vi "Initialize 8 NEO Swerve Drive.vi"() -> (0 "error out":errorcluster, 3 "Motors":T1={"Drive Motors (NEO)"={"Left Front"={"DeviceStatus"={"status"=FALSE, "code"=0, "source"=""}, "Type"=enum."PWM", "PWM"={"PWM Channel"=enum."Invalid", "DeadBand"={"Name"="", "maxPositivePwm"=0, "minPositivePwm"=0, "centerPwm"=0, "maxNegativePwm"=0, "minNegativePwm"=0, "angularRange"=0}}, "CAN"={"Device Number"=0, "SetOutput VI Ref"=variant, "GetOutput VI Ref"=variant, "Enable VI Ref"=variant, "Disable VI Ref"=variant, "Data"=variant}, "Invert"=FALSE, "DIO PWM"={"PWM \"Enable\" Channel"=enum."Invalid", "DIOChannel"=enum."Invalid", "PWM Rate"=0.0}}, "Left Back"={"DeviceStatus"={"status"=FALSE, "code"=0, "source"=""}, "Type"=enum."PWM", "PWM"={"PWM Channel"=enum."Invalid", "DeadBand"={"Name"="", "maxPositivePwm"=0, "minPositivePwm"=0, "centerPwm"=0, "maxNegativePwm"=0, "minNegativePwm"=0, "angularRange"=0}}, "CAN"={"Device Number"=0, "SetOutput VI Ref"=variant, "GetOutput VI Ref"=variant, "Enable VI Ref"=variant, "Disable VI Ref"=variant, "Data"=variant}, "Invert"=FALSE, "DIO PWM"={"PWM \"Enable\" Channel"=enum."Invalid", "DIOChannel"=enum."Invalid", "PWM Rate"=0.0}}, "Right Front"={"DeviceStatus"={"status"=FALSE, "code"=0, "source"=""}, "Type"=enum."PWM", "PWM"={"PWM Channel"=enum."Invalid", "DeadBand"={"Name"="", "maxPositivePwm"=0, "minPositivePwm"=0, "centerPwm"=0, "maxNegativePwm"=0, "minNegativePwm"=0, "angularRange"=0}}, "CAN"={"Device Number"=0, "SetOutput VI Ref"=variant, "GetOutput VI Ref"=variant, "Enable VI Ref"=variant, "Disable VI Ref"=variant, "Data"=variant}, "Invert"=FALSE, "DIO PWM"={"PWM \"Enable\" Channel"=enum."Invalid", "DIOChannel"=enum."Invalid", "PWM Rate"=0.0}}, "Right Back"={"DeviceStatus"={"status"=FALSE, "code"=0, "source"=""}, "Type"=enum."PWM", "PWM"={"PWM Channel"=enum."Invalid", "DeadBand"={"Name"="", "maxPositivePwm"=0, "minPositivePwm"=0, "centerPwm"=0, "maxNegativePwm"=0, "minNegativePwm"=0, "angularRange"=0}}, "CAN"={"Device Number"=0, "SetOutput VI Ref"=variant, "GetOutput VI Ref"=variant, "Enable VI Ref"=variant, "Disable VI Ref"=variant, "Data"=variant}, "Invert"=FALSE, "DIO PWM"={"PWM \"Enable\" Channel"=enum."Invalid", "DIOChannel"=enum."Invalid", "PWM Rate"=0.0}}}, "Steer Motors (NEO)"={"Left Front"={"DeviceStatus"={"status"=FALSE, "code"=0, "source"=""}, "Type"=enum."PWM", "PWM"={"PWM Channel"=enum."Invalid", "DeadBand"={"Name"="", "maxPositivePwm"=0, "minPositivePwm"=0, "centerPwm"=0, "maxNegativePwm"=0, "minNegativePwm"=0, "angularRange"=0}}, "CAN"={"Device Number"=0, "SetOutput VI Ref"=variant, "GetOutput VI Ref"=variant, "Enable VI Ref"=variant, "Disable VI Ref"=variant, "Data"=variant}, "Invert"=FALSE, "DIO PWM"={"PWM \"Enable\" Channel"=enum."Invalid", "DIOChannel"=enum."Invalid", "PWM Rate"=0.0}}, "Left Back"={"DeviceStatus"={"status"=FALSE, "code"=0, "source"=""}, "Type"=enum."PWM", "PWM"={"PWM Channel"=enum."Invalid", "DeadBand"={"Name"="", "maxPositivePwm"=0, "minPositivePwm"=0, "centerPwm"=0, "maxNegativePwm"=0, "minNegativePwm"=0, "angularRange"=0}}, "CAN"={"Device Number"=0, "SetOutput VI Ref"=variant, "GetOutput VI Ref"=variant, "Enable VI Ref"=variant, "Disable VI Ref"=variant, "Data"=variant}, "Invert"=FALSE, "DIO PWM"={"PWM \"Enable\" Channel"=enum."Invalid", "DIOChannel"=enum."Invalid", "PWM Rate"=0.0}}, "Right Front"={"DeviceStatus"={"status"=FALSE, "code"=0, "source"=""}, "Type"=enum."PWM", "PWM"={"PWM Channel"=enum."Invalid", "DeadBand"={"Name"="", "maxPositivePwm"=0, "minPositivePwm"=0, "centerPwm"=0, "maxNegativePwm"=0, "minNegativePwm"=0, "angularRange"=0}}, "CAN"={"Device Number"=0, "SetOutput VI Ref"=variant, "GetOutput VI Ref"=variant, "Enable VI Ref"=variant, "Disable VI Ref"=variant, "Data"=variant}, "Invert"=FALSE, "DIO PWM"={"PWM \"Enable\" Channel"=enum."Invalid", "DIOChannel"=enum."Invalid", "PWM Rate"=0.0}}, "Right Back"={"DeviceStatus"={"status"=FALSE, "code"=0, "source"=""}, "Type"=enum."PWM", "PWM"={"PWM Channel"=enum."Invalid", "DeadBand"={"Name"="", "maxPositivePwm"=0, "minPositivePwm"=0, "centerPwm"=0, "maxNegativePwm"=0, "minNegativePwm"=0, "angularRange"=0}}, "CAN"={"Device Number"=0, "SetOutput VI Ref"=variant, "GetOutput VI Ref"=variant, "Enable VI Ref"=variant, "Disable VI Ref"=variant, "Data"=variant}, "Invert"=FALSE, "DIO PWM"={"PWM \"Enable\" Channel"=enum."Invalid", "DIOChannel"=enum."Invalid", "PWM Rate"=0.0}}}, "Pigeon2"={"DeviceStatus"={"status"=FALSE, "code"=0, "source"=""}, "Device Number"=0, "Type"=352321536, "Device ID"=0, "Handle"=0, "UsageFrame"=0, "Library Path"=path ""}, "Radii (ft)"={"Left Front Position"=[], "Left Back Position"=[], "Right Front Position"=[], "Right Back Position"=[]}} {"Radii (ft)"."Right Back Position" format="%.2f"; "Radii (ft)"."Right Front Position" format="%.2f"; "Radii (ft)"."Left Back Position" format="%.2f"; "Radii (ft)"."Left Front Position" format="%.2f"; "Pigeon2"."Type" items=["CAN"=352321536, "TalonSRX"=33554432]})   [LabVIEW 2025]
doc: "Creates a cluster of 4 motors (order is left-front, left-back, right-front, right-back) initialized with PID coefficients and status frame reduction"
uses:
  <vilib>/Rock Robotics/WPI/ThirdParty/REV Robotics/REVLib/Typedef/Spark MAX Idle Mode.ctl
  <vilib>/Rock Robotics/WPI/MotorControl/WPI_MotorControlType.ctl
  <vilib>/Rock Robotics/SystemInterfaces/DIO/FPGA_DIOPWMChannel.ctl
  <vilib>/Rock Robotics/WPI/PWM/WPI_PWMDeadband.ctl
  <vilib>/Rock Robotics/SystemInterfaces/DIO/FPGA_DIOChannel.ctl
  <vilib>/Rock Robotics/WPI/MotorControl/WPI_MotorControlDeviceRef.ctl
  Type Definitions/Hardware/4 Motor Sets/(NEO & NEO 550) 4 Motor Set.ctl
  Type Definitions/Hardware/Swerve Drives/(NEO-NEO-ThroughBore-Pigeon2) Swerve.ctl
  Type Definitions/Data/Pod Positions.ctl
  <vilib>/Rock Robotics/WPI/ThirdParty/Phoenix-LabVIEW/Pigeon IMU/CTRE_PigeonIMU_ConnectionType.ctl
  <vilib>/Rock Robotics/WPI/ThirdParty/Phoenix-LabVIEW/Pigeon IMU/CTRE_PigeonIMU_DeviceRef.ctl
  Type Definitions/Hardware/Swerve Configs/NEO-NEO-ThroughBore-Pigeon2 Swerve Config.ctl
  <vilib>/Rock Robotics/WPI/ThirdParty/REV Robotics/REVLib/SubVI/Public/SPARK Open Brushless.vi
  <vilib>/Rock Robotics/WPI/ThirdParty/REV Robotics/REVLib/Typedef/Spark MAX Status Frames.ctl
  <vilib>/Rock Robotics/WPI/ThirdParty/REV Robotics/REVLib/Typedef/Closed Loop Voltage Mode.ctl
  <vilib>/Rock Robotics/WPI/ThirdParty/REV Robotics/REVLib/Typedef/SPARK Feedback Sensor.ctl
  <vilib>/Rock Robotics/WPI/ThirdParty/REV Robotics/REVLib/SubVI/Public/SPARK Configure Encoder Conversion Factors.vi
  <vilib>/Rock Robotics/WPI/ThirdParty/REV Robotics/REVLib/SubVI/Public/SPARK Configure Power Smart Current Limit.vi
  <vilib>/Rock Robotics/WPI/ThirdParty/REV Robotics/REVLib/SubVI/Public/SPARK Configure Basic Idle Mode.vi
  <vilib>/Rock Robotics/WPI/ThirdParty/REV Robotics/REVLib/SubVI/Public/SPARK Configure Closed Loop Voltage Mode.vi
  <vilib>/Rock Robotics/WPI/ThirdParty/REV Robotics/REVLib/SubVI/Public/SPARK Configure Closed Loop Basic.vi
  <vilib>/Rock Robotics/WPI/ThirdParty/REV Robotics/REVLib/SubVI/Public/SPARK Configure Closed Loop Position Wrapping.vi
  <vilib>/Rock Robotics/WPI/ThirdParty/REV Robotics/REVLib/SubVI/Public/SPARK Configure Encoder Velocity Filtering UVW.vi
  <vilib>/Rock Robotics/WPI/ThirdParty/REV Robotics/REVLib/Typedef/Spark MAX Hall Sensor Average Depth Size.ctl
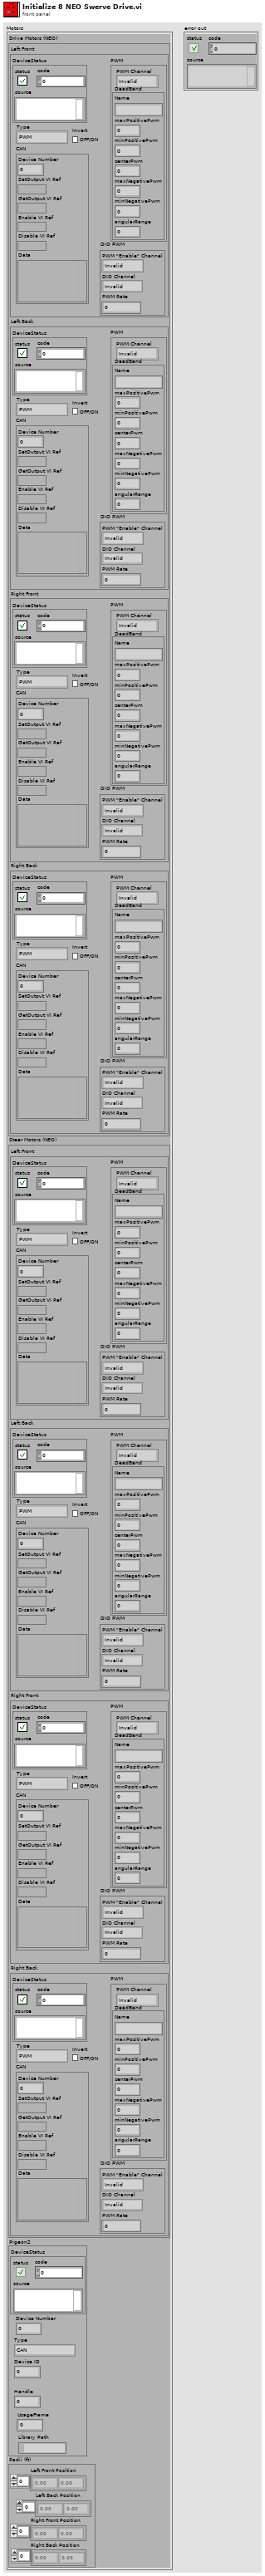
[diagram p1: front panel]
types:
  T1 = typedef "(NEO-NEO-ThroughBore-Pigeon2) Swerve.ctl" = cluster{"Drive Motors (NEO)":T2, "Steer Motors (NEO)":T2, "Pigeon2":T8, "Radii (ft)":T10}
  T2 = typedef "(NEO & NEO 550) 4 Motor Set.ctl" = cluster{"Left Front":T3, "Left Back":T3, "Right Front":T3, "Right Back":T3}
  T3 = typedef "WPI_MotorControlDeviceRef.ctl" = cluster{"DeviceStatus":errorcluster, "Type":T4, "PWM":cluster{"PWM Channel":T5, "DeadBand":T6}, "CAN":cluster{"Device Number":u8, "SetOutput VI Ref":variant, "GetOutput VI Ref":variant, "Enable VI Ref":variant, "Disable VI Ref":variant, "Data":variant}, "Invert":bool, "DIO PWM":cluster{"PWM \"Enable\" Channel":T5, "DIOChannel":T7, "PWM Rate":dbl}}
  T4 = typedef "WPI_MotorControlType.ctl" = enum16{"PWM", "CAN", "DIO PWM"}
  T5 = typedef "FPGA_DIOPWMChannel.ctl" = enum8{"PWM 0", "PWM 1", "PWM 2", "PWM 3", "PWM 4", "PWM 5", "PWM 6", "PWM 7", "PWM 8", "PWM 9", "PWM MXP 0", "PWM MXP 1", "PWM MXP 2", "PWM MXP 3", "PWM MXP 4", "PWM MXP 5", "PWM MXP 6", "PWM MXP 7", "PWM MXP 8", "PWM MXP 9", "Invalid"}
  T6 = typedef "WPI_PWMDeadband.ctl" = cluster{"Name":string, "maxPositivePwm":i32, "minPositivePwm":i32, "centerPwm":i32, "maxNegativePwm":i32, "minNegativePwm":i32, "angularRange":u16}
  T7 = typedef "FPGA_DIOChannel.ctl" = enum8{"DIO 0", "DIO 1", "DIO 2", "DIO 3", "DIO 4", "DIO 5", "DIO 6", "DIO 7", "DIO 8", "DIO 9", "DIO MXP 0", "DIO MXP 1", "DIO MXP 2", "DIO MXP 3", "DIO MXP 4", "DIO MXP 5", "DIO MXP 6", "DIO MXP 7", "DIO MXP 8", "DIO MXP 9", "DIO MXP 10", "DIO MXP 11", "DIO MXP 12", "DIO MXP 13", "DIO MXP 14", "DIO MXP 15", "SPI Port CS1", "SPI Port CS2", "SPI Port CS3", "SPI Port MISO", "SPI Port MOSI", "Invalid"}
  T8 = typedef "CTRE_PigeonIMU_DeviceRef.ctl" = cluster{"DeviceStatus":errorcluster, "Device Number":u8, "Type":T9, "Device ID":u32, "Handle":u64, "UsageFrame":u32, "Library Path":path}
  T9 = typedef "CTRE_PigeonIMU_ConnectionType.ctl" = u32
  T10 = typedef "Pod Positions.ctl" = cluster{"Left Front Position":dbl[], "Left Back Position":dbl[], "Right Front Position":dbl[], "Right Back Position":dbl[]}
  T11 = typedef "NEO-NEO-ThroughBore-Pigeon2 Swerve Config.ctl" = cluster{"Drive Motor CAN IDs":cluster{"LF CAN ID":dbl, "LB CAN ID":dbl, "RF CAN ID":dbl, "RB CAN ID":dbl}, "Steer Motor CAN IDs":cluster{"LF CAN ID":dbl, "LB CAN ID":dbl, "RF CAN ID":dbl, "RB CAN ID":dbl}, "Drive PID Constants":cluster{"P Gain":dbl, "I Gain":dbl, "D Gain":dbl, "F Gain":dbl, "I Zone":dbl, "Min Output":dbl, "Max Output":dbl}, "Steer PID Constants":cluster{"P Gain":dbl, "I Gain":dbl, "D Gain":dbl, "F Gain":dbl, "I Zone":dbl, "Min Output":dbl, "Max Output":dbl}, "Pigeon 2 Refnum":string, "Pod Locations (ft)":T10}
  T12 = cluster{"LF CAN ID":dbl, "LB CAN ID":dbl, "RF CAN ID":dbl, "RB CAN ID":dbl}
  T13 = cluster{"P Gain":dbl, "I Gain":dbl, "D Gain":dbl, "F Gain":dbl, "I Zone":dbl, "Min Output":dbl, "Max Output":dbl}
  T14 = typedef "Spark MAX Hall Sensor Average Depth Size.ctl" = enum16{"1", "2", "4", "8"}
  T15 = typedef "SPARK Feedback Sensor.ctl" = enum16{"No Sensor", "Primary Encoder", "Analog Sensor", "Alternate or External Encoder", "Duty Cycle Sensor"}
  T16 = typedef "Closed Loop Voltage Mode.ctl" = enum16{"Disabled", "Voltage Output", "Voltage Compensation"}
  T17 = typedef "Spark MAX Status Frames.ctl" = enum16{"Status 0", "Status 1", "Status 2", "Status 3", "Status 4", "Status 5", "Status 6", "Status 7"}
  T18 = typedef "Spark MAX Idle Mode.ctl" = enum16{"Coast", "Brake"}
  T19 = typedef "DeviceReference.ctl" = cluster{"CANbus Name":string, "Device Encoding":u32, "Device Name":string}
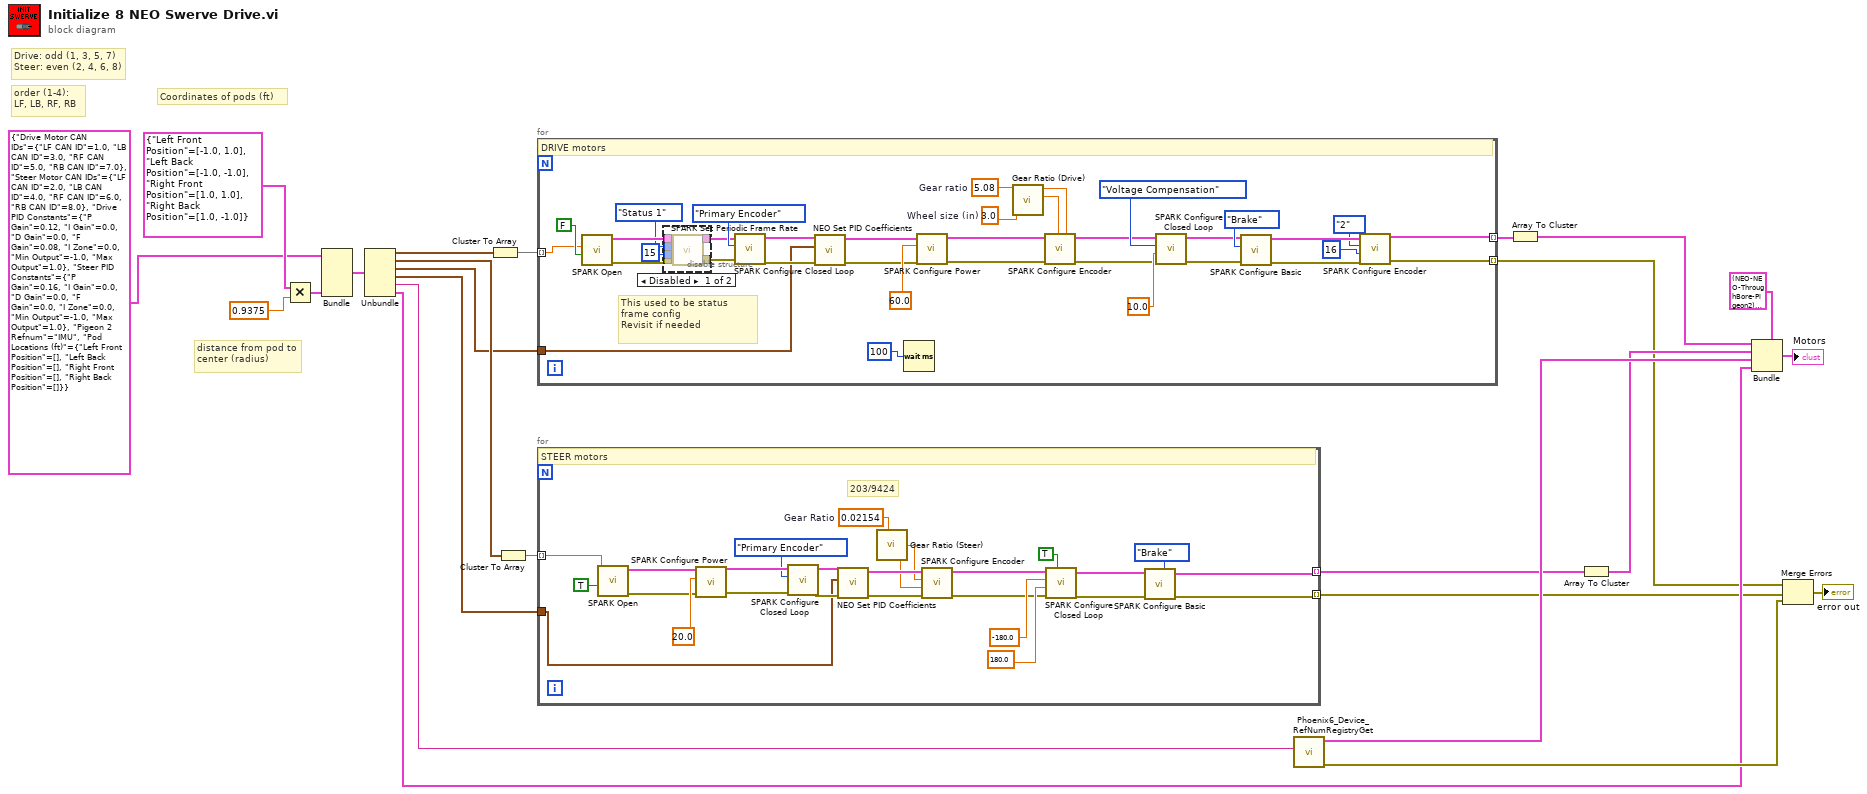
[diagram p0: block diagram]
diagram:
  # "Drive: odd (1, 3, 5, 7)\nSteer: even (2, 4, 6, 8)"
  # "Coordinates of pods (ft)"
  # "distance from pod to center (radius)"
  # "order (1-4):\nLF, LB, RF, RB"
  n1 = Multiply(x=T10 {"Left Front Position"=[-1.0, 1.0], "Left Back Position"=[-1.0, -1.0], "Right Front Position"=[1.0, 1.0], "Right Back Position"=[1.0, -1.0]} ("Radii (ft)"), y=0.9375 ("Pod Radius")) -> (x*y=w11:T10)
  n2 = Bundle(cluster=T11 {"Drive Motor CAN IDs"={"LF CAN ID"=1.0, "LB CAN ID"=3.0, "RF CAN ID"=5.0, "RB CAN ID"=7.0}, "Steer Motor CAN IDs"={"LF CAN ID"=2.0, "LB CAN ID"=4.0, "RF CAN ID"=6.0, "RB CAN ID"=8.0}, "Drive PID Constants"={"P Gain"=0.12, "I Gain"=0.0, "D Gain"=0.0, "F Gain"=0.08, "I Zone"=0.0, "Min Output"=-1.0, "Max Output"=1.0}, "Steer PID Constants"={"P Gain"=0.16, "I Gain"=0.0, "D Gain"=0.0, "F Gain"=0.0, "I Zone"=0.0, "Min Output"=-1.0, "Max Output"=1.0}, "Pigeon 2 Refnum"="IMU", "Pod Locations (ft)"={"Left Front Position"=[], "Left Back Position"=[], "Right Front Position"=[], "Right Back Position"=[]}} ("Swerve Config"), "Pod Locations (ft)"=w11) -> (w20:T11)  [unwired: 5 in]
  n3 = Unbundle(w20) -> ("Drive Motor CAN IDs"=w19:T12, "Steer Motor CAN IDs"=w18:T12, "Drive PID Constants"=w15:T13, "Steer PID Constants"=w14:T13, "Pigeon 2 Refnum"=w13:string, "Pod Locations (ft)"=w12:T10)
  n4 = Cluster To Array(cluster=w19) -> (array=w24:dbl[])
  n5 = Cluster To Array(cluster=w18) -> (array=w23:dbl[])
  n6 = for {
    tunnel: w24 -> [w33] mode=indexing
    tunnel: w15 -> [w26]
    tunnel: [w32] -> w6 mode=indexing
    tunnel: [w31] -> w2 mode=indexing
    w53 = 3.0  # Wheel size (in)
    w56 = 5.08  # Gear ratio
    # "This used to be status frame config\nRevisit if needed"
    # "DRIVE motors"
    n7 = call-poly <vilib>:"SPARK Open.vi"("Invert"=FALSE, "Device Number"=w33) -> ("error out"=w57:errorcluster, "MotorControlDeviceRef"=w58:T3)  [unwired: 8 in]
    n8 = disable-structure shown="Disabled" {
      disable-tunnel: w58 -> [w63 w65]
      disable-tunnel: w57 -> [w62 w64]
      disable-tunnel: u16 15 ("Frame rate (ms)") -> [w61 _]
      disable-tunnel: Spark_MAX_Status_Frames."Status 1" ("Frame") -> [w60 _]
      disable-tunnel: [_ w65] -> w37
      disable-tunnel: [_ w64] -> w36
      frame Disabled {
        n9 = call <vilib>:"SPARK Set Periodic Frame Rate.vi"("error in"=w62, "Frame rate (ms)"=w61, "Frame"=w60, "MotorControlDeviceRef"=w63) -> ()  [unwired: 6 in, 2 out]
      }
      frame Enabled {
      }
    }
    n10 = call-poly <vilib>:"SPARK Configure Closed Loop.vi"("error in"=w36, "Feedback Sensor (Primary Encoder)"=SPARK_Feedback_Sensor."Primary Encoder", "MotorControlDeviceRef in"=w37) -> ("error out"=w27:errorcluster, "MotorControlDeviceRef out"=w30:T3)  [unwired: 7 in]
    n11 = call "NEO Set PID Coefficients.vi"("error in"=w27, "PID Constants"=w26, "MotorControlDeviceRef in"=w30) -> ("error out"=w28:errorcluster, "MotorControlDeviceRef out"=w29:T3)  [unwired: 5 in]
    n12 = Wait (ms)(milliseconds to wait=u32 100) -> ()  [unwired: 1 out]
    n13 = call-poly <vilib>:"SPARK Configure Power.vi"("error in (no error)"=w28, "Primay Current Limit (80A)"=60.0, "MotorControlDeviceRef in"=w29) -> ("error out"=w41:errorcluster, "MotorControlDeviceRef out"=w42:T3)  [unwired: 7 in]
    n14 = call "Gear Ratio (Drive).vi"("Wheel size (in)"=w53, "Gear ratio"=w56) -> ("Position Factor"=w54:dbl, "Velocity Factor (ft/s)"=w55:dbl)  [unwired: 8 in]
    n15 = call-poly <vilib>:"SPARK Configure Encoder.vi"("error in"=w41, "Velocity Conversion Factor"=w55, "Position Conversion Factor"=w54, "MotorControlDeviceRef in"=w42) -> ("error out"=w43:errorcluster, "MotorControlDeviceRef out"=w44:T3)  [unwired: 6 in]
    n16 = call-poly <vilib>:"SPARK Configure Closed Loop.vi"("error in (no error)"=w43, "Compensated Nominal Voltage"=10.0 ("Nominal Voltage"), "Voltage Mode (Disabled)"=Closed_Loop_Voltage_Mode."Voltage Compensation", "MotorControlDeviceRef in"=w44) -> ("error out"=w45:errorcluster, "MotorControlDeviceRef out"=w46:T3)  [unwired: 6 in]
    n17 = call-poly <vilib>:"SPARK Configure Basic.vi"("error in (no error)"=w45, "Idle Mode"=Spark_MAX_Idle_Mode."Brake", "MotorControlDeviceRef in"=w46) -> ("error out"=w39:errorcluster, "MotorControlDeviceRef out"=w40:T3)  [unwired: 7 in]
    n18 = call-poly <vilib>:"SPARK Configure Encoder.vi"("error in"=w39, "Measurement Period (ms)"=u32 16, "Average Depth (8)"=Spark_MAX_Hall_Sensor_Average_Depth_Size."2", "MotorControlDeviceRef in"=w40) -> ("error out"=w31:errorcluster, "MotorControlDeviceRef out"=w32:T3)  [unwired: 6 in]
  }
  n19 = for {
    tunnel: w23 -> [w91] mode=indexing
    tunnel: w14 -> [w69]
    tunnel: [w78] -> w4 mode=indexing
    tunnel: [w77] -> w3 mode=indexing
    w66 = 0.02154  # Gear Ratio
    # "203/9424"
    # "STEER motors"
    n20 = call-poly <vilib>:"SPARK Open.vi"("Invert"=TRUE, "Device Number"=w91) -> ("error out"=w79:errorcluster, "MotorControlDeviceRef"=w80:T3)  [unwired: 8 in]
    n21 = call-poly <vilib>:"SPARK Configure Power.vi"("error in (no error)"=w79, "Primay Current Limit (80A)"=20.0, "MotorControlDeviceRef in"=w80) -> ("error out"=w71:errorcluster, "MotorControlDeviceRef out"=w72:T3)  [unwired: 7 in]
    n22 = call-poly <vilib>:"SPARK Configure Closed Loop.vi"("error in"=w71, "Feedback Sensor (Primary Encoder)"=SPARK_Feedback_Sensor."Primary Encoder", "MotorControlDeviceRef in"=w72) -> ("error out"=w73:errorcluster, "MotorControlDeviceRef out"=w76:T3)  [unwired: 7 in]
    n23 = call "NEO Set PID Coefficients.vi"("error in"=w73, "PID Constants"=w69, "MotorControlDeviceRef in"=w76) -> ("error out"=w74:errorcluster, "MotorControlDeviceRef out"=w75:T3)  [unwired: 5 in]
    n24 = call "Gear Ratio (Steer).vi"("Gear Ratio"=w66) -> ("Position Factor"=w68:dbl, "Velocity Factor"=w67:dbl)  [unwired: 6 in]
    n25 = call-poly <vilib>:"SPARK Configure Encoder.vi"("error in"=w74, "Velocity Conversion Factor"=w67, "Position Conversion Factor"=w68, "MotorControlDeviceRef in"=w75) -> ("error out"=w81:errorcluster, "MotorControlDeviceRef out"=w82:T3)  [unwired: 6 in]
    n26 = call-poly <vilib>:"SPARK Configure Closed Loop.vi"("Enable (T)"=TRUE ("Enable (F)"), "error in"=w81, "Maximum Input"=180.0 ("Maximum Output (0)"), "Minimum Input"=-180.0 ("Minimum Input (0)"), "MotorControlDeviceRef in"=w82) -> ("error out"=w83:errorcluster, "MotorControlDeviceRef out"=w84:T3)  [unwired: 5 in]
    n27 = call-poly <vilib>:"SPARK Configure Basic.vi"("error in (no error)"=w83, "Idle Mode"=Spark_MAX_Idle_Mode."Brake", "MotorControlDeviceRef in"=w84) -> ("error out"=w77:errorcluster, "MotorControlDeviceRef out"=w78:T3)  [unwired: 7 in]
  }
  n28 = call <vilib>:"Phoenix6_Device_RefNumRegistryGet.vi"("refnum name"=w13) -> ("error out"=w17:errorcluster, "data"=w7:T19)  [unwired: 9 in]
  n29 = Array To Cluster(array=w6) -> (cluster=w1:cluster{"[0]":T3, "[1]":T3, "[2]":T3, "[3]":T3})
  n30 = Array To Cluster(array=w4) -> (cluster=w5:cluster{"[0]":T3, "[1]":T3, "[2]":T3, "[3]":T3})
  n31 = Bundle(cluster=T1 {"Drive Motors (NEO)"={"Left Front"={"DeviceStatus"={"status"=FALSE, "code"=0, "source"=""}, "Type"=enum."PWM", "PWM"={"PWM Channel"=enum."Invalid", "DeadBand"={"Name"="", "maxPositivePwm"=0, "minPositivePwm"=0, "centerPwm"=0, "maxNegativePwm"=0, "minNegativePwm"=0, "angularRange"=0}}, "CAN"={"Device Number"=0, "SetOutput VI Ref"=variant, "GetOutput VI Ref"=variant, "Enable VI Ref"=variant, "Disable VI Ref"=variant, "Data"=variant}, "Invert"=FALSE, "DIO PWM"={"PWM \"Enable\" Channel"=enum."Invalid", "DIOChannel"=enum."Invalid", "PWM Rate"=0.0}}, "Left Back"={"DeviceStatus"={"status"=FALSE, "code"=0, "source"=""}, "Type"=enum."PWM", "PWM"={"PWM Channel"=enum."Invalid", "DeadBand"={"Name"="", "maxPositivePwm"=0, "minPositivePwm"=0, "centerPwm"=0, "maxNegativePwm"=0, "minNegativePwm"=0, "angularRange"=0}}, "CAN"={"Device Number"=0, "SetOutput VI Ref"=variant, "GetOutput VI Ref"=variant, "Enable VI Ref"=variant, "Disable VI Ref"=variant, "Data"=variant}, "Invert"=FALSE, "DIO PWM"={"PWM \"Enable\" Channel"=enum."Invalid", "DIOChannel"=enum."Invalid", "PWM Rate"=0.0}}, "Right Front"={"DeviceStatus"={"status"=FALSE, "code"=0, "source"=""}, "Type"=enum."PWM", "PWM"={"PWM Channel"=enum."Invalid", "DeadBand"={"Name"="", "maxPositivePwm"=0, "minPositivePwm"=0, "centerPwm"=0, "maxNegativePwm"=0, "minNegativePwm"=0, "angularRange"=0}}, "CAN"={"Device Number"=0, "SetOutput VI Ref"=variant, "GetOutput VI Ref"=variant, "Enable VI Ref"=variant, "Disable VI Ref"=variant, "Data"=variant}, "Invert"=FALSE, "DIO PWM"={"PWM \"Enable\" Channel"=enum."Invalid", "DIOChannel"=enum."Invalid", "PWM Rate"=0.0}}, "Right Back"={"DeviceStatus"={"status"=FALSE, "code"=0, "source"=""}, "Type"=enum."PWM", "PWM"={"PWM Channel"=enum."Invalid", "DeadBand"={"Name"="", "maxPositivePwm"=0, "minPositivePwm"=0, "centerPwm"=0, "maxNegativePwm"=0, "minNegativePwm"=0, "angularRange"=0}}, "CAN"={"Device Number"=0, "SetOutput VI Ref"=variant, "GetOutput VI Ref"=variant, "Enable VI Ref"=variant, "Disable VI Ref"=variant, "Data"=variant}, "Invert"=FALSE, "DIO PWM"={"PWM \"Enable\" Channel"=enum."Invalid", "DIOChannel"=enum."Invalid", "PWM Rate"=0.0}}}, "Steer Motors (NEO)"={"Left Front"={"DeviceStatus"={"status"=FALSE, "code"=0, "source"=""}, "Type"=enum."PWM", "PWM"={"PWM Channel"=enum."Invalid", "DeadBand"={"Name"="", "maxPositivePwm"=0, "minPositivePwm"=0, "centerPwm"=0, "maxNegativePwm"=0, "minNegativePwm"=0, "angularRange"=0}}, "CAN"={"Device Number"=0, "SetOutput VI Ref"=variant, "GetOutput VI Ref"=variant, "Enable VI Ref"=variant, "Disable VI Ref"=variant, "Data"=variant}, "Invert"=FALSE, "DIO PWM"={"PWM \"Enable\" Channel"=enum."Invalid", "DIOChannel"=enum."Invalid", "PWM Rate"=0.0}}, "Left Back"={"DeviceStatus"={"status"=FALSE, "code"=0, "source"=""}, "Type"=enum."PWM", "PWM"={"PWM Channel"=enum."Invalid", "DeadBand"={"Name"="", "maxPositivePwm"=0, "minPositivePwm"=0, "centerPwm"=0, "maxNegativePwm"=0, "minNegativePwm"=0, "angularRange"=0}}, "CAN"={"Device Number"=0, "SetOutput VI Ref"=variant, "GetOutput VI Ref"=variant, "Enable VI Ref"=variant, "Disable VI Ref"=variant, "Data"=variant}, "Invert"=FALSE, "DIO PWM"={"PWM \"Enable\" Channel"=enum."Invalid", "DIOChannel"=enum."Invalid", "PWM Rate"=0.0}}, "Right Front"={"DeviceStatus"={"status"=FALSE, "code"=0, "source"=""}, "Type"=enum."PWM", "PWM"={"PWM Channel"=enum."Invalid", "DeadBand"={"Name"="", "maxPositivePwm"=0, "minPositivePwm"=0, "centerPwm"=0, "maxNegativePwm"=0, "minNegativePwm"=0, "angularRange"=0}}, "CAN"={"Device Number"=0, "SetOutput VI Ref"=variant, "GetOutput VI Ref"=variant, "Enable VI Ref"=variant, "Disable VI Ref"=variant, "Data"=variant}, "Invert"=FALSE, "DIO PWM"={"PWM \"Enable\" Channel"=enum."Invalid", "DIOChannel"=enum."Invalid", "PWM Rate"=0.0}}, "Right Back"={"DeviceStatus"={"status"=FALSE, "code"=0, "source"=""}, "Type"=enum."PWM", "PWM"={"PWM Channel"=enum."Invalid", "DeadBand"={"Name"="", "maxPositivePwm"=0, "minPositivePwm"=0, "centerPwm"=0, "maxNegativePwm"=0, "minNegativePwm"=0, "angularRange"=0}}, "CAN"={"Device Number"=0, "SetOutput VI Ref"=variant, "GetOutput VI Ref"=variant, "Enable VI Ref"=variant, "Disable VI Ref"=variant, "Data"=variant}, "Invert"=FALSE, "DIO PWM"={"PWM \"Enable\" Channel"=enum."Invalid", "DIOChannel"=enum."Invalid", "PWM Rate"=0.0}}}, "Pigeon2"={"DeviceStatus"={"status"=FALSE, "code"=0, "source"=""}, "Device Number"=0, "Type"=352321536, "Device ID"=0, "Handle"=0, "UsageFrame"=0, "Library Path"=path ""}, "Radii (ft)"={"Left Front Position"=[], "Left Back Position"=[], "Right Front Position"=[], "Right Back Position"=[]}} ("(N-N-C-P) Swerve Motors"), "Drive Motors (NEO)"=w1, "Steer Motors (NEO)"=w5, "Pigeon2"=w7, "Radii (ft)"=w12) -> (→"Motors":T1)
  n32 = Merge Errors(w2, w3, w17) -> (→"error out":errorcluster)
